vi "History Update.vi"(8 "error in (no error)":errorcluster, 10 "History Record":T2, 11 "Connection Refnum":T1) -> (0 "error out":errorcluster, 3 "Connection Refnum":T1)   [LabVIEW 2011]
uses:
  History Record.ctl
  SI.LIB/ODBC/SQL Controls/Connection Refnum.ctl
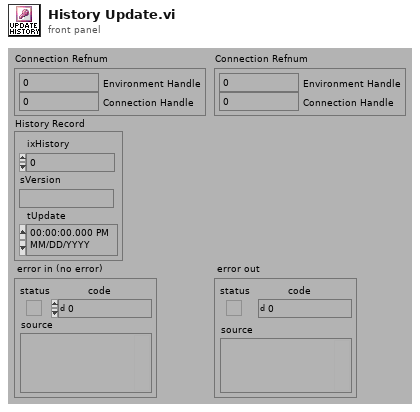
[diagram p1: front panel]
types:
  T1 = typedef "Connection Refnum.ctl" = cluster{"Environment Handle":i32, "Connection Handle":i32}
  T2 = typedef "History Record.ctl" = cluster{"ixHistory":i32, "sVersion":string, "tUpdate":timestamp}
  T3 = typedef "Statement Refnum.ctl" = cluster{"Statement Handle":i32, "Parameter Number":u16}
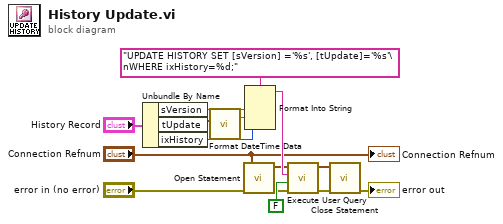
[diagram p0: block diagram]
diagram:
  n1 = Unbundle By Name("History Record") -> ("sVersion"=w9:string, "tUpdate"=w2:timestamp, "ixHistory"=w6:i32)
  n2 = call "Format DateTime Data.vi"("Timestamp in"=w2) -> ("UTC DB String out"=w1:string)  [unwired: 10 out]
  n3 = call "Open Statement.vi"("error in (no error)"="error in (no error)", "Connection Refnum"="Connection Refnum") -> ("error out"=w8:errorcluster, "Statement Refnum"=w7:T3)  [unwired: 4 out]
  n4 = Format Into String(format string="UPDATE HISTORY SET [sVersion] ='%s', [tUpdate]='%s'\nWHERE ixHistory=%d;" ("User Query"), w9, w1, w6) -> (resulting string=w10:string)  [unwired: 2 in, 1 out]
  n5 = call "Execute User Query.vi"("error in (no error)"=w8, "Return Data? (f)"=FALSE, "User Query"=w10, "Statement Refnum"=w7) -> ("error out"=w13:errorcluster, "Statement Refnum"=w12:T3)  [unwired: 2 out]
  n6 = call "Close Statement.vi"("error in (no error)"=w13, "Statement Refnum"=w12) -> ("error out"=→"error out":errorcluster)  [unwired: 5 out]
  "Connection Refnum" <- "Connection Refnum"
